vi "TCam_WellCalculater.vi"(6 "DrawTempOverlay":bool, 8 "Well Pos":T2[](array[typedef]) {"Y" format="%.2f"; "X" format="%.2f"}, 9 "Pixels":cluster{"X":i32, "Y":i32}[][](array[cluster]), 10 "Image in":T1, 11 "index":i32) -> (2 "Image Out":T1, 3 "mean":dbl format="%0.2f")   [LabVIEW 2021]
uses:
  <vilib>/vision/Image Controls.llb/IMAQ Image.ctl
  <vilib>/Analysis/baseanly.llb/Mean (DBL).vi
  <vilib>/vision/NI_Vision_Development_Module.lvlib
  <vilib>/Analysis/NI_AALBase.lvlib
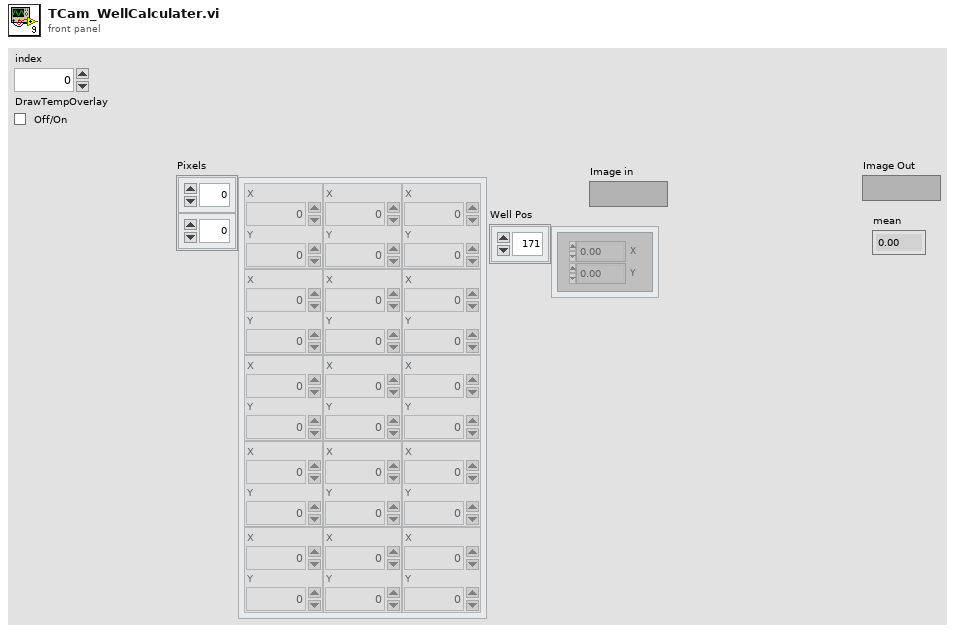
[diagram p1: front panel]
types:
  T1 = typedef "IMAQ Image.ctl" = refnum<image>
  T2 = typedef "IMAQ Point" = cluster{"X":sgl, "Y":sgl}
  T3 = cluster{"Desired Font (Application)":enum16{"User-specified Font", "Application Font", "System Font", "Dialog Font"}, "[User-specified Font]":cluster{"Font Name":string, "Size":i16, "Strikeout?":bool, "Italic?":bool, "Underline?":bool, "Outline?":bool, "Shadow?":bool, "Bold?":bool, "Rotation Angle":dbl}, "Horizontal Alignment":i16, "Vertical Alignment":i16}
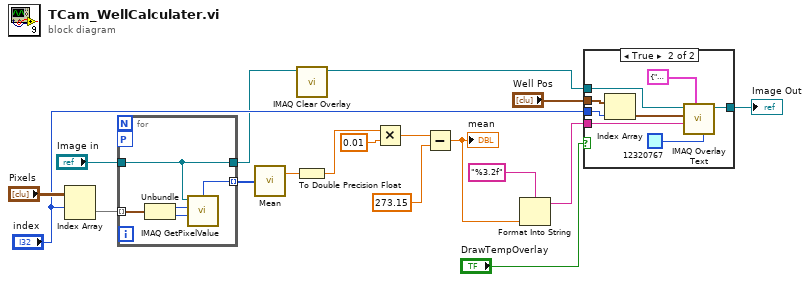
[diagram p0: block diagram]
diagram:
  n1 = Index Array(array="Pixels", index (row)="index") -> (element=w13:cluster{"X":i32, "Y":i32}[])  [unwired: 1 in]
  n2 = for {
    tunnel: "Image in" -> [w20]
    tunnel: w13 -> [w23] mode=indexing
    tunnel: [w19] -> w12 mode=indexing
    tunnel: [w20] -> w9
    workers-P: _ -> [_]
    n3 = Unbundle(w23) -> ("X"=w22:i32, "Y"=w21:i32)
    n4 = call "IMAQ GetPixelValue"("Image"=w20, "X Coordinate"=w22, "Y Coordinate"=w21) -> ("Pixel Value (U16)"=w19:u16)  [unwired: 3 in, 4 out]
  }
  n5 = call-poly <vilib>:"Mean.vi"("X"=w12) -> ("mean"=w3:dbl)  [unwired: 1 out]
  n6 = call "IMAQ Clear Overlay"("Image"=w9) -> ("Image Out"=w8:T1)  [unwired: 9 in, 1 out]
  n7 = To Double Precision Float(number=w3) -> (double precision float=w5:dbl)
  n8 = Multiply(x=w5, y=0.01) -> (x*y=w6:dbl)
  n9 = Subtract(x=w6, y=273.15) -> (x-y=w2:dbl)
  "mean" <- w2
  n10 = Format Into String(format string="%3.2f", w2) -> (resulting string=w10:string)  [unwired: 2 in, 1 out]
  n11 = case shown="True" "DrawTempOverlay" {
    tunnel: [w24 w32] -> w17
    tunnel: "Well Pos" -> [_ w31]
    tunnel: "index" -> [_ w29]
    tunnel: w10 -> [_ w27]
    tunnel: w8 -> [w24 w25]
    frame False {
    }
    frame True {
      n12 = Index Array(array=w31, index=w29) -> (element=w30:T2)
      n13 = call "IMAQ Overlay Text"("BG Color (Transparent)"=u32 12320767, "Font, Size & Style"=T3 {"Desired Font (Application)"=enum."Application Font", "[User-specified Font]"={"Font Name"="", "Size"=6, "Strikeout?"=FALSE, "Italic?"=FALSE, "Underline?"=FALSE, "Outline?"=FALSE, "Shadow?"=FALSE, "Bold?"=FALSE, "Rotation Angle"=0.0}, "Horizontal Alignment"=1, "Vertical Alignment"=0}, "String"=w27, "Origin"=w30, "Image"=w25) -> ("Image Out"=w32:T1)  [unwired: 5 in, 1 out]
    }
  }
  "Image Out" <- w17
